vi "Main.vi"() -> ()   [LabVIEW 2020]
uses:
  Public/Controls/CCW button.ctl
  Public/Controls/CW button.ctl
  States -- typedef.ctl
  Public/Controls/Motor info.ctl
  Public/Controls/Move motor parameters--cluster.ctl
  Public/Controls/Motor direction.ctl
  Public/Controls/Step style.ctl
  Public/Controls/Com Port Options.ctl
  Public/Controls/Motor initialization parameters--cluster.ctl
  951c27e0-d3ae-4342-ab9a-27cd7722bbe2.vi
  0e09bd5c-b6a7-474e-9505-972206d0d40d.vi
  Public/Write--init.vi
  Public/Write--move.vi
  Public/Write--home.vi
  <vilib>/regexp/Match Regular Expression.xnode
  Control de MaP.lvlib
panel:
  out "Comando(string) 2":string
  in  "stop":bool
  in  "Go to zero":bool
  in  "Set zero":bool
  out "Angulo inicial":dbl caption="Ángulo \nActual M1"
  in  "Velocidad del motor\n(0-255)":u16=100
  out "Ready":bool caption="Arduino ready"
  out "Save":bool caption="Guardando datos"
  in  "Ángulo final":dbl=90.0
  out "Angulo M2":dbl caption="Ángulo \nActual M2" format="%#_3g°"
  out "Angulo M1":dbl caption="Ángulo \nActual M1" format="%#_3g°"
  out "0° M2":bool
  out "0° M1":bool
  in  "RESOLUCIÓN":dbl=1.0 caption="Avance" format="%#_g°"
  in  "CW Button M1":T1
  in  "CCW Button M1":T2
  in  "CCW Button M2":T1
  in  "CW Button M2":T2
  in  "Tab Control":T3(tab)
  out "Valor de Sensor":dbl(slide) scale=0.0..1.0
  in  "Intensidad del Láser":u8(slide) step=1 scale=0.0..255.0
  in  "Read sensor":bool
  out "Real Time Measurement":cluster{"X":dbl, "Y":dbl}[](graph)
  in  "Realizar Análisis":bool
  in  "Abrir Archivo":path
  in  "q Final":dbl=80.0
  in  "q Inicial":dbl=40.0
  out "No. de Muestras":i32
  out "Ancho de Curva":dbl format="%#.3g"
  out "Intensidad \nMáxima":dbl
  out "qR":dbl
  out "Intensidad \nMínima":dbl
  out "q Medio":dbl
  out "Brewster Angle Analysis":cluster{"EJE X":dbl[], dbl[]}(graph)
  out "Índice":dbl
  in  "Abeles Brewster":bool
  in  "Abrir Archivo de Sustrato":path
  in  "Abrir Archivo de Película":path
  in  "calcular error":bool
  out "Abeles Brewster Analysis":cluster{dbl[], dbl[]}[](graph)
  in  "q Inicial 2":dbl=40.0
  in  "q Final  2":dbl=80.0
  out "Película qB":dbl
  out "Película qB +error":dbl
  in  "Error (Grados)":dbl
  out "Sustrato qB":dbl
  out "Sustrato IR":dbl format="%#.4g"
  out "Película IR":dbl format="%#.4g"
  out "ángulo B medio":dbl
  out "Película IR +error":dbl format="%#.4g"
  in  "Home":bool
  out "Recibo de Datos":string
  in  "Get all info":bool
  in  "Read End-stops":bool
  in  "Get position":bool
  out "Idle":bool
  in  "Stop motors":bool
  in  "Move motors":bool
  # "Programa: Control de motores a pasos \npara medición de ángulo de Brewster y \ntécnica de Abelès-Brewster"
  # "Desarrollado por: Oscar Javier Silva Hernández &\nDiego Torres Armenta"
  # "Controles Manuales y Automáticos"
  # "MOTOR 1"
  # "MOTOR 2"
  # "Información del sistema"
  # "¡ATENCIÓN! Lea estas instrucciones y recomendaciones antes de operar el programa.\nEste programa ejecuta el control manual y automático del sistema en general.\nUna vez que se haya elegido el puerto COM donde tenemos ubicada nuestra tarjeta de adquisición de datos, el programa inicializará con un protocolo de calibración de motores. NO PRESIONE NINGÚN BOTÓN.\nDe manera automática el programa moverá las platinas rotatorias al ángulo 0°. Una vez que los indicadores 0° M1 y 0° M2 estén encendidos, el indicador del Ángulo Actual M1 se habilitará y el podremos iniciar a operar el programa."
  # "Controles Manuales y Automáticos (Controladores e Indicadores)\n\n-MOTOR 1 & 2: Para ambos motores se tiene un botón de movimiento hacia adelante y otro botón de movimiento hacia atrás indicado con flechas. Durante el reinicio de posición 0°, el botón hacia atrás se deshabilita para evitar conflictos mecánicos.\n-0° M1 & 0° M2: Indicadores de posición 0° para ambos motores.\n-FIN: Indica si se está terminó de realizar un movimiento.\n-Ángulo Actual M1 & M2: Muestra la posición actual para cada motor.\n-RESOLUCIÓN: Valor de grados definido por el usuario para realizar movimientos manuales de manera independiente para cada motor. Es utilizado para alinear el sistema con respecto al láser antes y después de realizar mediciones.\n-Reiniciar Posición: Inicia el protocolo de reinicio de posición para regresar los motores a 0°.\n-Mover y Guardar: Se inicia el barrido ángular desde la posición actual de los motores hasta la posición indicada en el controlador Barrido Angular.\n-Cancelar: Cancela cualquier movimiento o instrucción que se esté ejecutando. My útil para detener instrucciones y cerrar el programa sin tener conflictos."
  # "Parámetros iniciales & Información (Controladores e Indicadores)\n\n-SALIR: Cerramos el programa una vez que hayamos terminado de utilizarlo. Es importante no presionar este botón en medio de un movimiento de motor o alguna otra instrucción.\n-Pantalla: Toda la información generada por los eventos de usuario es mostrada en esta pantalla.\n-Programa habilitado: Se enciende cuando el proceso de inicialización se realiza exitosamente y el programa queda listo para operar.\n-Guardar Datos: Indica si los datos están siendo capturados durante el barrido angular."
  # "Gráfica, Ángulo de Brewster & Abelès-Brewster Analysis\n\n-Gráfica: Esta sección es utilizada para llevar a cabo las mediciones. Dentro podemos encontrar un indicador del valor de la intensidad de la luz capturada por el sensor, un controlador para la intensidad de la luz de salida del láser semiconductor.\n-Ángulo de Brewster: En esta sección podemos realizar el análisis de ángulo de Brewster de mediciones realizadas por el sistema para encontrar los parámetros característicos de la curva. Seleccionamos el archivo deseado, definimos el ángulo inicial y final y presionamos el botón ANALISIS.\n-Abelès-Brewster: Muy similar a la sección anterior, podemos realizar el ánalisis de Abelès-Brewster de mediciones realizadas para sustratos con y sin película delgada. También podemos calcular el error del resultado."
  # "Montura de\nSustratos"
  # "Ensamble \nde Motores"
  # "Montura \nde Prismas"
  # "Sistema Completo con Montura de Sustratos"
  # "Ensamble de Láser con Polarizador"
  # "Sistema Completo con Montura de Prismas"
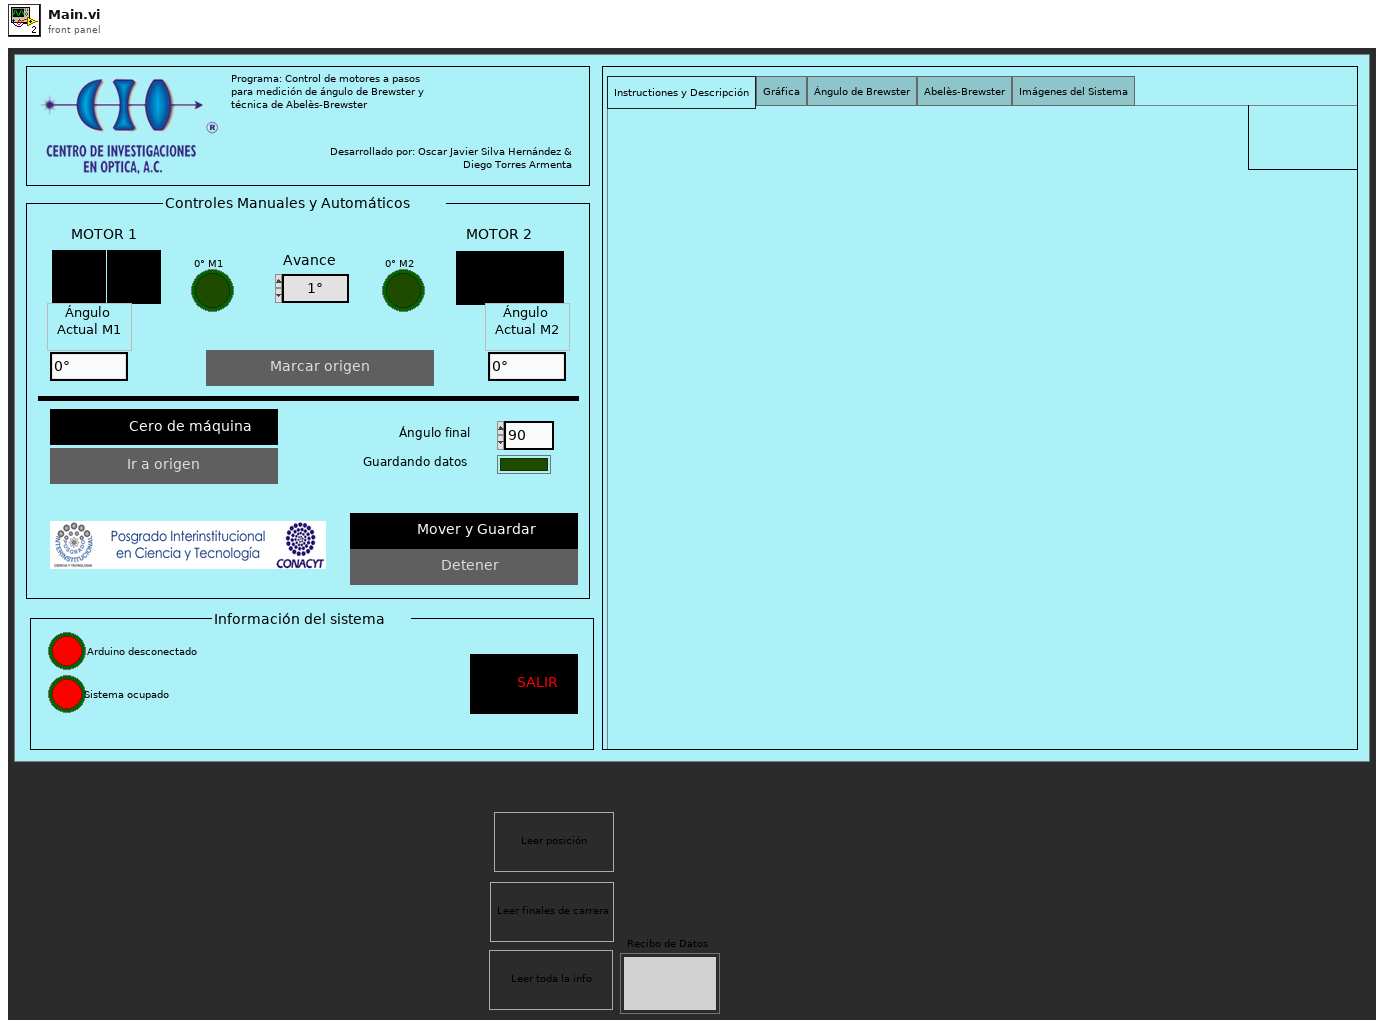
[diagram p1: front panel]
types:
  T1 = typedef "CW button.ctl" = bool
  T2 = typedef "CCW button.ctl" = bool
  T3 = enum32{"Instructiones y Descripción", "Gráfica", "Ángulo de Brewster", "Abelès-Brewster", "Imágenes del Sistema"}
  T4 = cluster{"refnum out":refnum<file>, "path":path, "path string":string}
  T5 = typedef "Control de MaP.lvlib/Motor info.ctl" = cluster{"Motor positions":dbl[], "Sensor value":dbl, "End-stop state":bool[], "°/step":dbl[], "Motor params":T6, "Moving?":bool, "Home?":bool, "Connected?":bool, "Manual zero?":bool}
  T6 = typedef "Control de MaP.lvlib/Move motor parameters--cluster.ctl" = cluster{"Action":u8, "Direction motor 1":T7, "Direction motor 2":T7, "Steps motor 1":u16, "Steps motor 2":u16, "Step style motor 1":T8, "Step style motor 2":T8}
  T7 = typedef "Control de MaP.lvlib/Motor direction.ctl" = u8
  T8 = typedef "Control de MaP.lvlib/Step style.ctl" = u8
  T9 = typedef "States -- typedef.ctl" = enum16{"Initilaize", "Update FP", "Enable/disable controls", "Wait", "Update config", "Configuration dialog", "Exit", "Init motor"}
  T10 = typedef "Config -- cluster.ctl" = cluster{"Arduino port":refnum<visa-resource-name>, "Starting angle M1":dbl, "Starting angle M2":dbl}
  T11 = enum8{"Enabled", "Disabled", "Disabled and Grayed Out"}
  T12 = typedef "Control de MaP.lvlib/Motor initialization parameters--cluster.ctl" = cluster{"Action":u8, "Steps per rev motor 1":u8, "Steps per rev motor 2":u8, "RPM motor 1":u16, "RPM motor 2":u16}
  T13 = typedef "Control de MaP.lvlib/Com Port Options.ctl" = cluster{"baud rate (9600)":u32, "data bits (8)":u16, "parity (0:none)":enum16{"None", "Odd", "Even", "Mark", "Space"}}
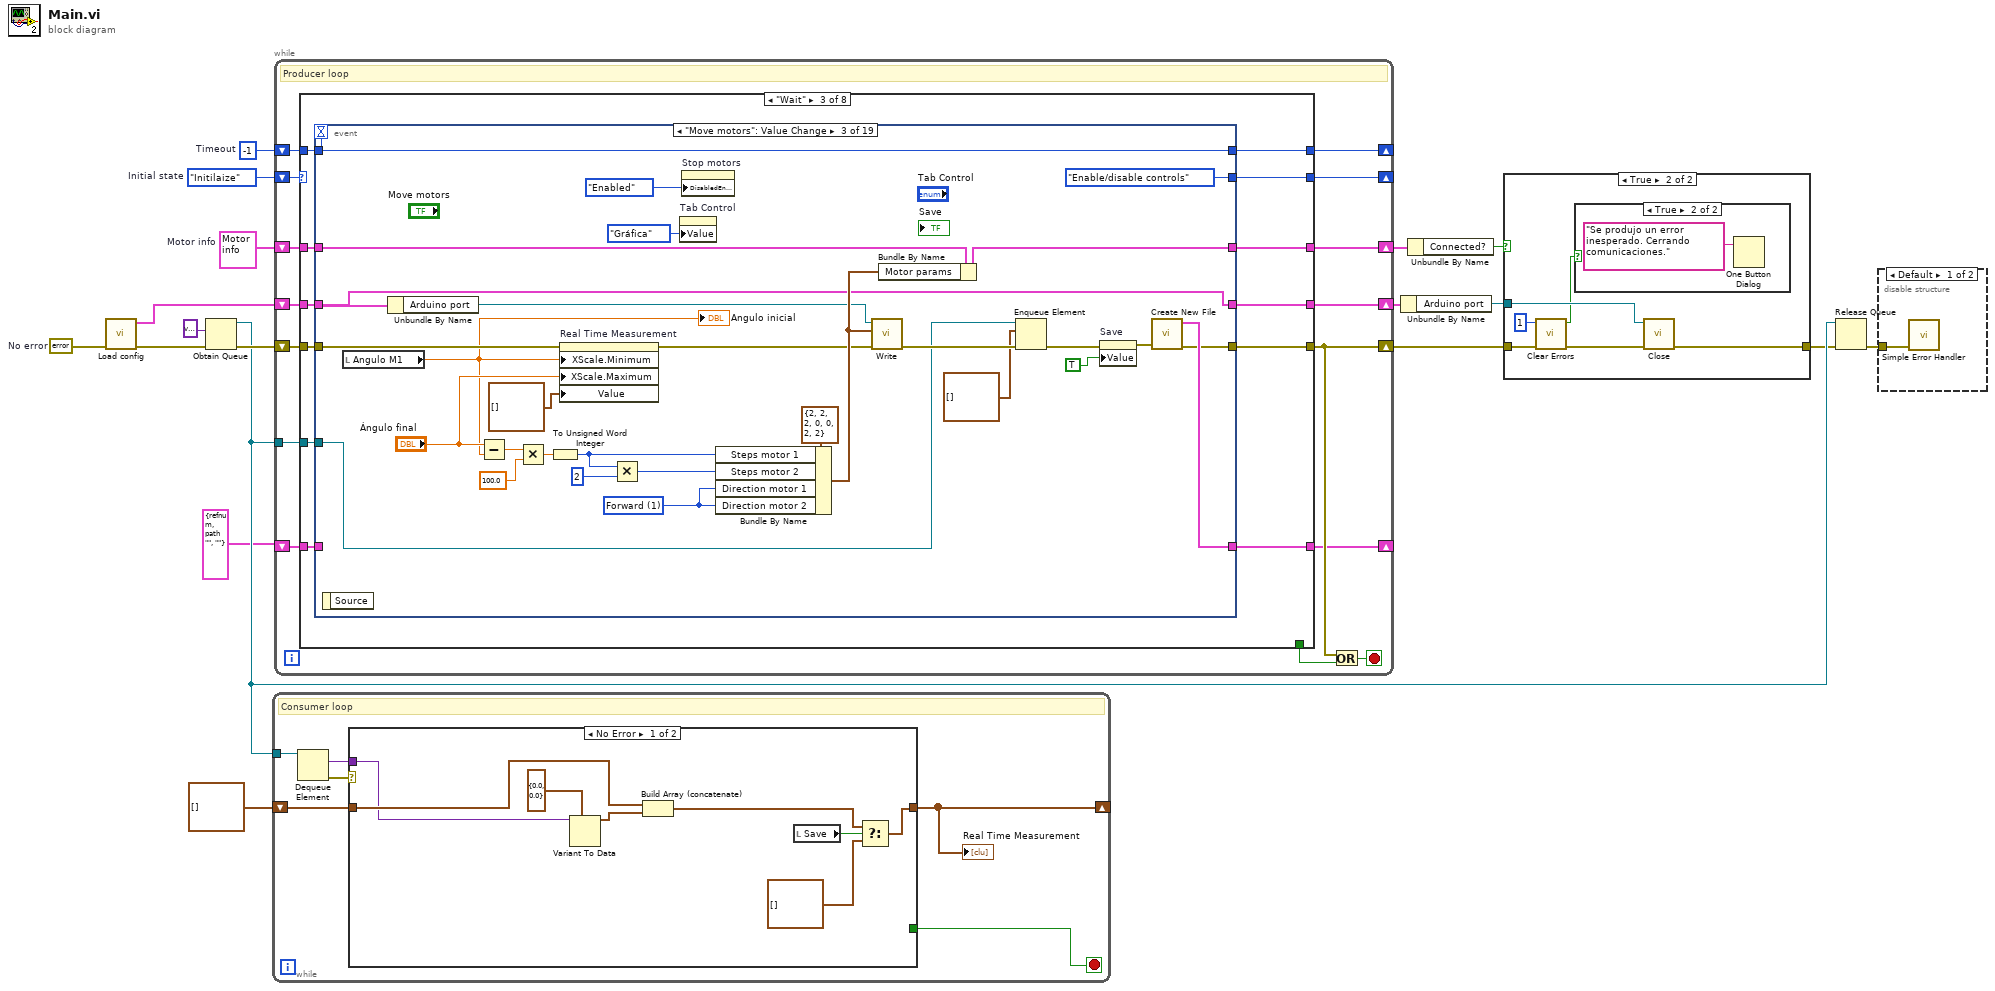
[diagram p0: block diagram]
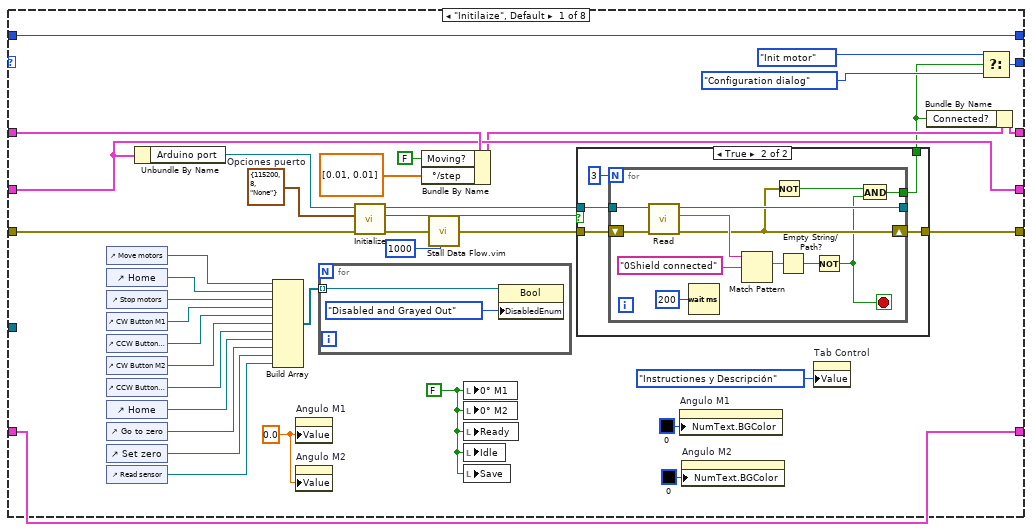
[diagram p2: hidden frame]
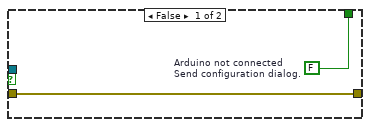
[diagram p3: hidden frame]
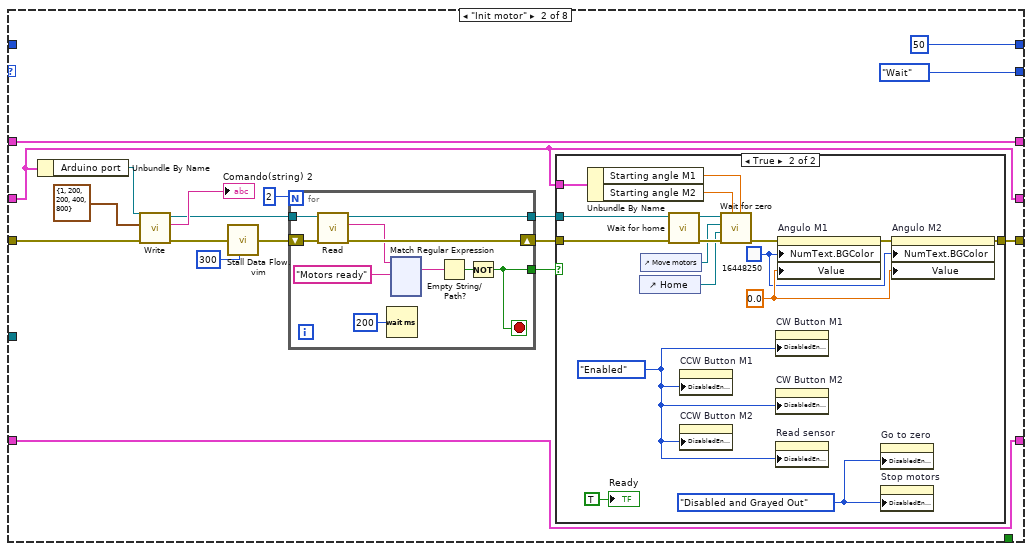
[diagram p4: hidden frame]
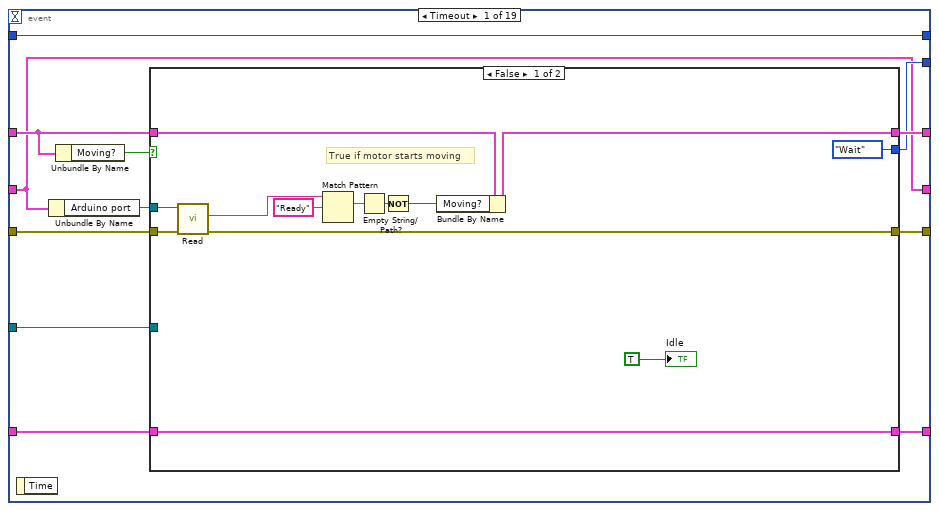
[diagram p6: hidden frame]
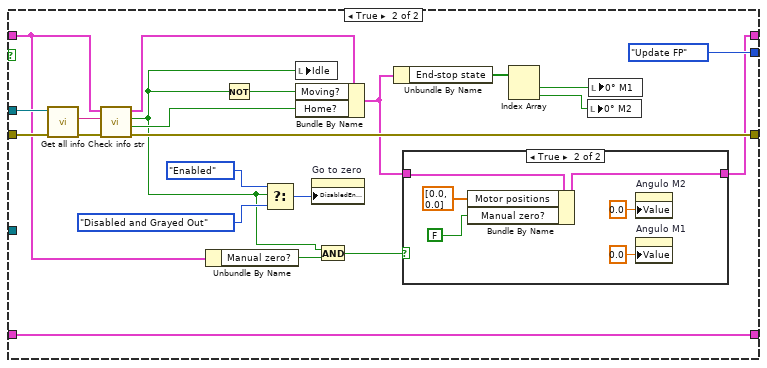
[diagram p7: hidden frame]
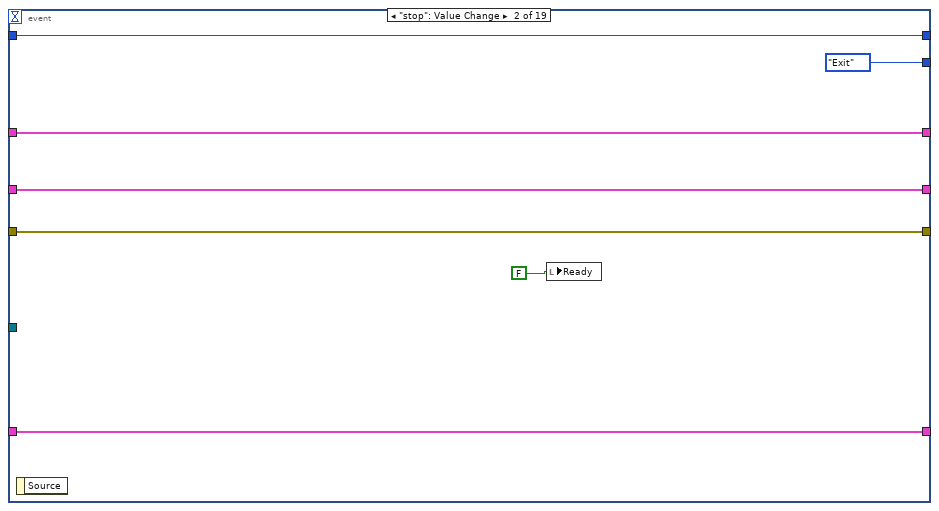
[diagram p9: hidden frame]
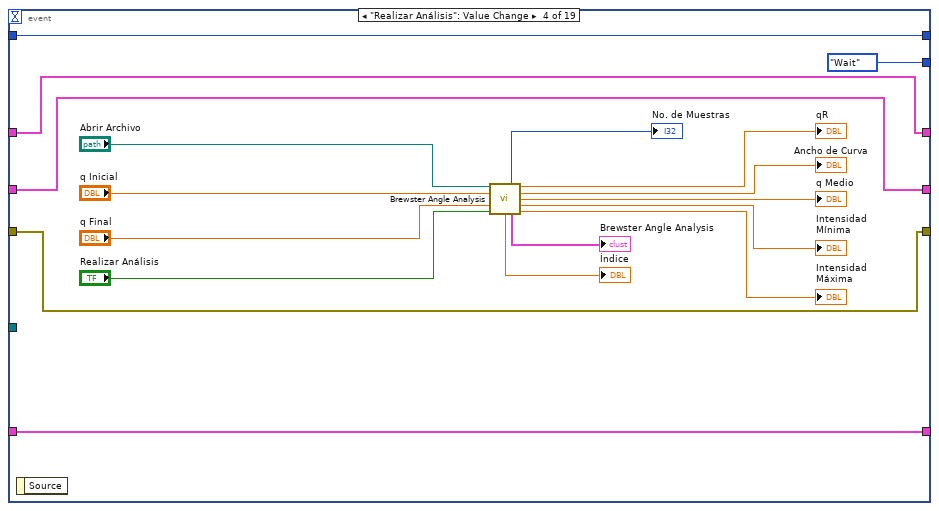
[diagram p10: hidden frame]
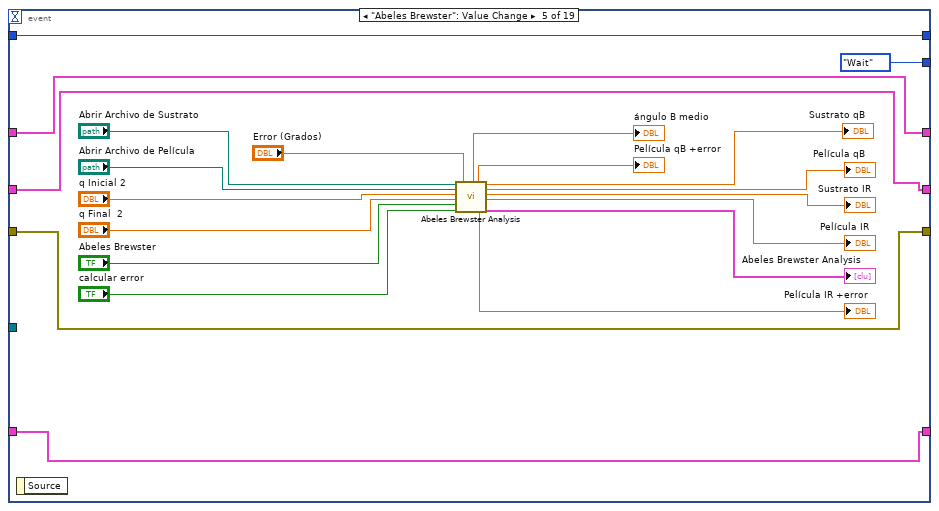
[diagram p11: hidden frame]
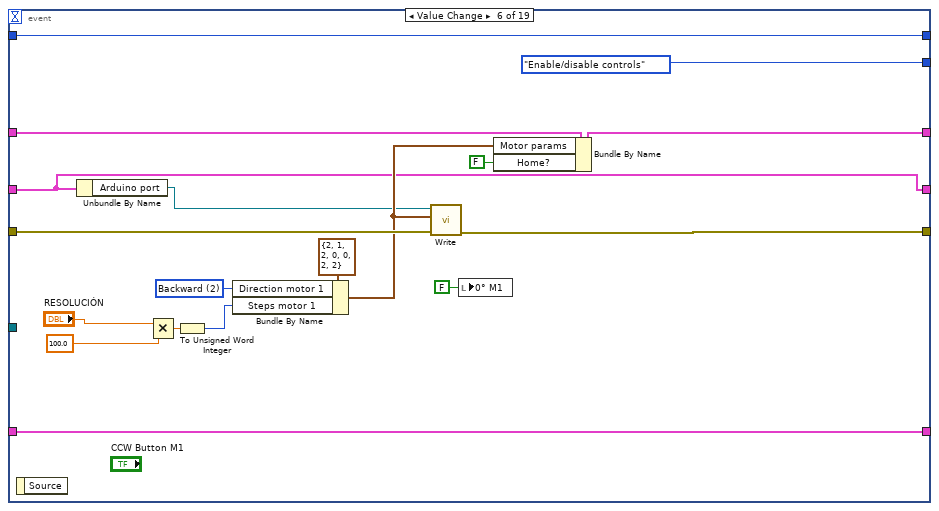
[diagram p12: hidden frame]
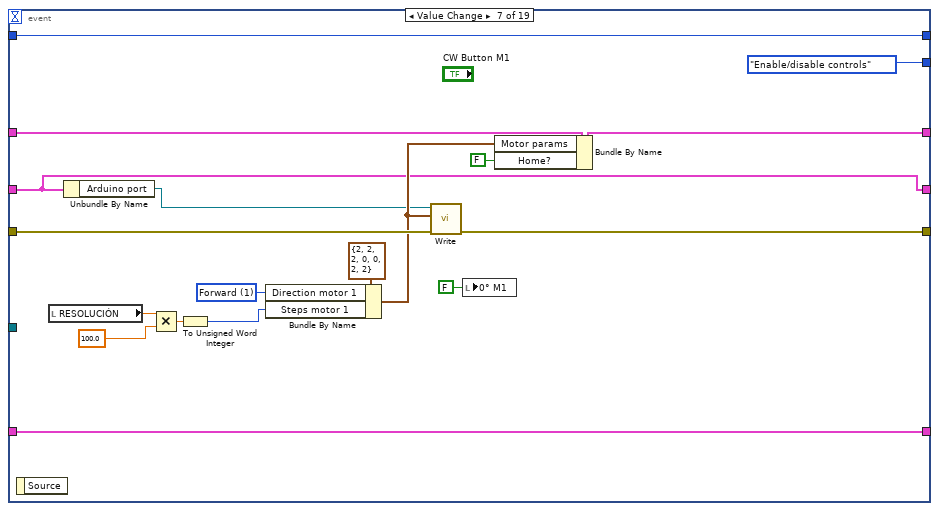
[diagram p13: hidden frame]
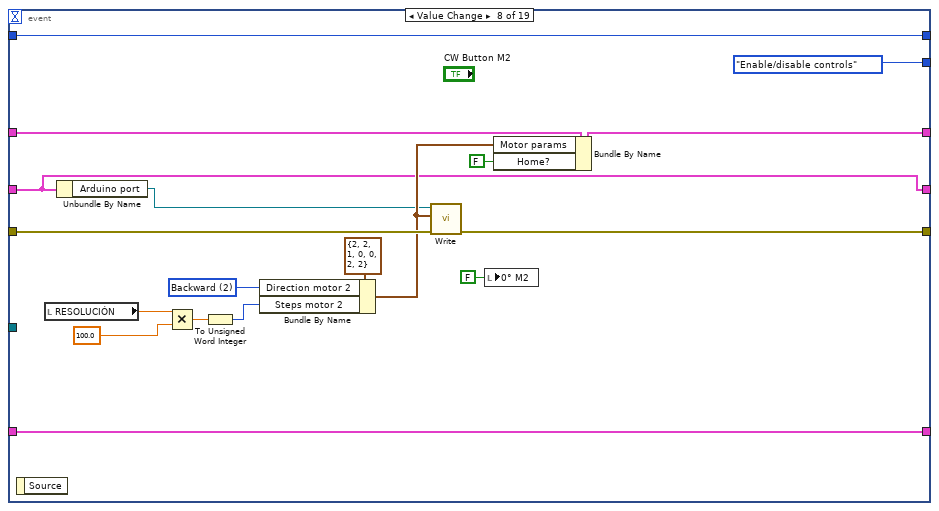
[diagram p14: hidden frame]
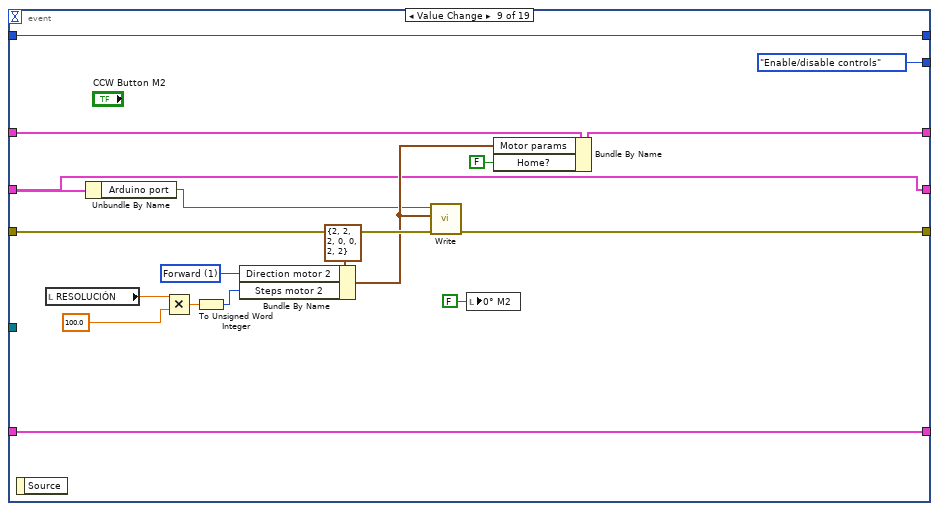
[diagram p15: hidden frame]
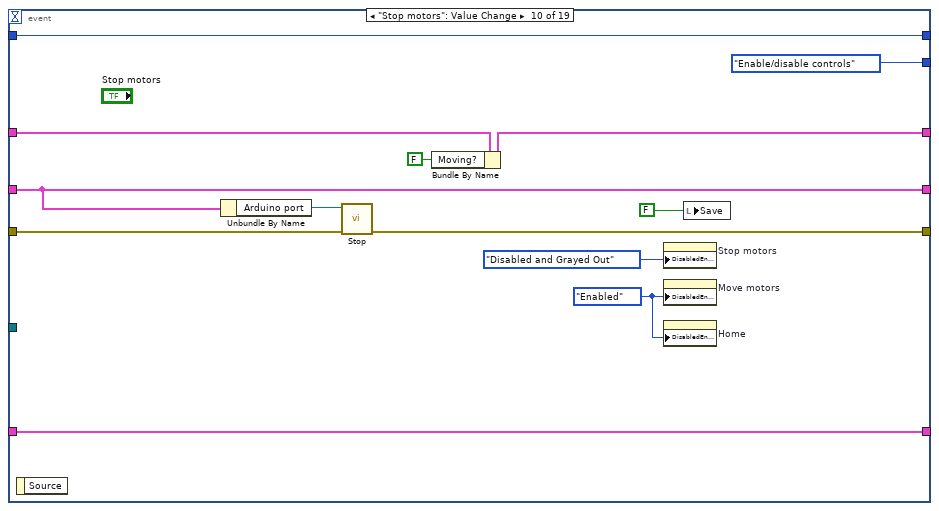
[diagram p16: hidden frame]
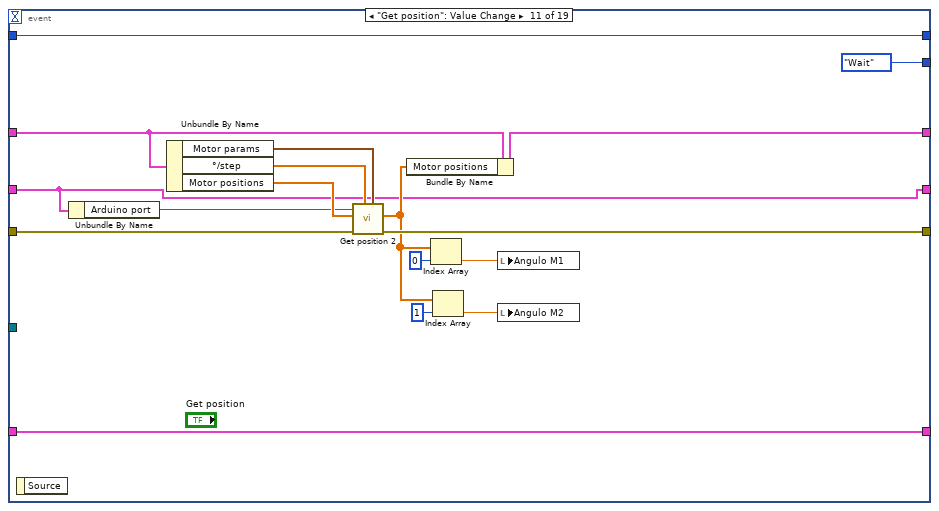
[diagram p17: hidden frame]
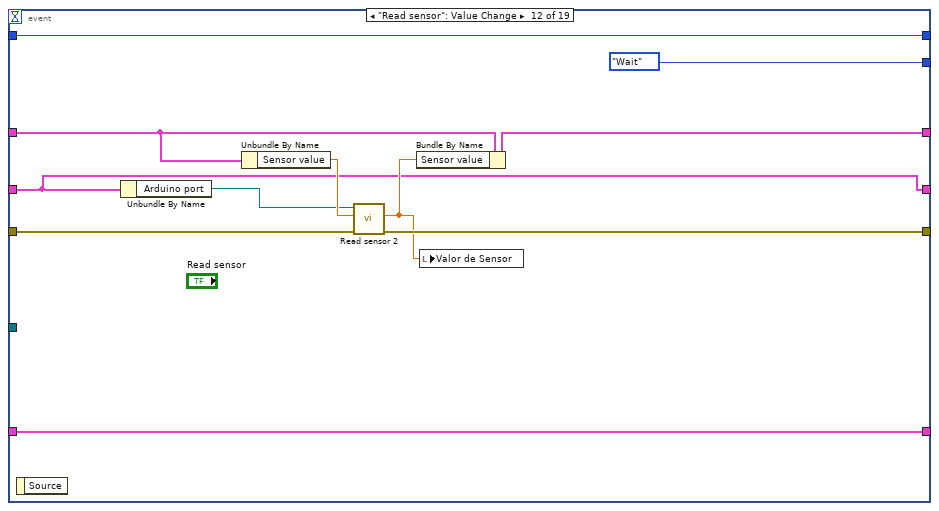
[diagram p18: hidden frame]
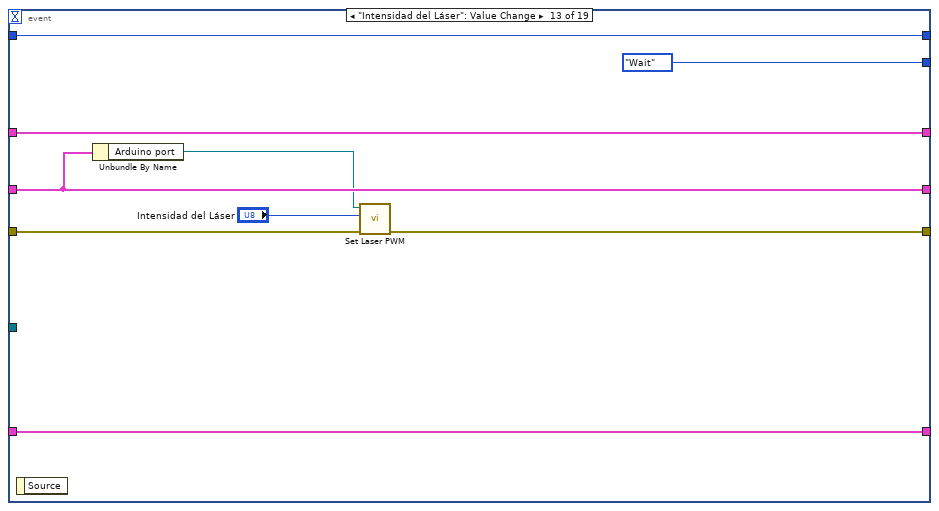
[diagram p19: hidden frame]
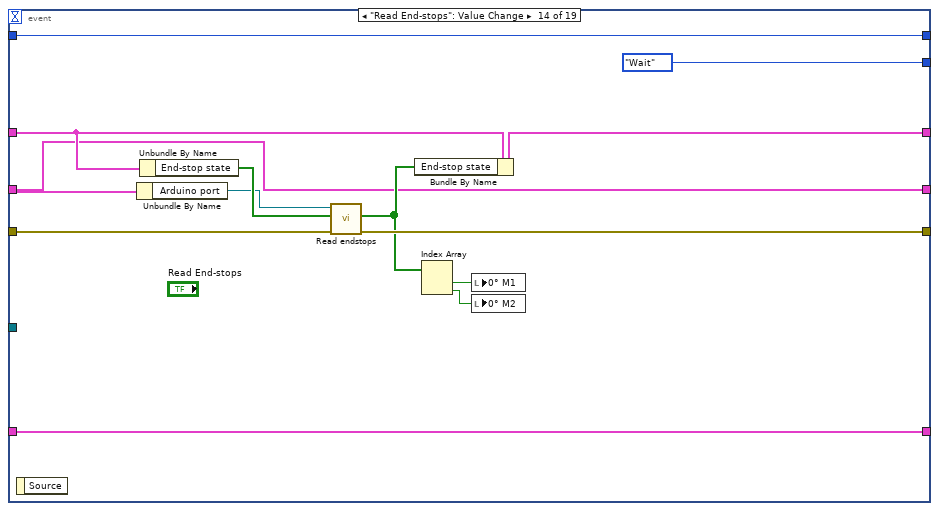
[diagram p20: hidden frame]
diagram:
  w15 = T5 {"Motor positions"=[0.0, 0.0], "Sensor value"=0.0, "End-stop state"=[FALSE, FALSE], "°/step"=[], "Motor params"={"Action"=2, "Direction motor 1"=1, "Direction motor 2"=1, "Steps motor 1"=100, "Steps motor 2"=100, "Step style motor 1"=1, "Step style motor 2"=1}, "Moving?"=FALSE, "Home?"=FALSE, "Connected?"=FALSE, "Manual zero?"=FALSE}  # Motor info
  w16 = -1  # Timeout
  w4 = errorcluster {"status"=FALSE, "code"=0, "source"=""}  # No error
  w18 = States_--_typedef."Initilaize"  # Initial state
  n1 = call "Load config.vi"("error in (no error)"=w4) -> ("error out"=w3:errorcluster, "Config"=w5:T10)  [unwired: 9 in]
  n2 = Obtain Queue(element data type=variant, error in (no error)=w3) -> (queue out=w11:refnum<queue>, error out=w13:errorcluster)  [unwired: 3 in, 1 out]
  n3 = while {
    tunnel: w11 -> [w24]
    shift-right: [w19] -> _
    shift-left: cluster{"Ángulo M1":dbl, "Voltage":dbl}[] [] ("cluster") -> [w23]
    stop <- w20 stop-if-true
    # "Consumer loop"
    n4 = Dequeue Element(queue=w24) -> (element=w22:variant, error out=w21:errorcluster)  [unwired: 2 in, 2 out]
    n5 = case shown="No Error" w21 {
      tunnel: w23 -> [w32 _]
      tunnel: w22 -> [w31 _]
      tunnel: [w26 cluster{"Ángulo M1":dbl, "Voltage":dbl}[] [] ("cluster")] -> w19
      tunnel: [_ TRUE] -> w20
      frame No Error {
        n6 = Variant To Data(type=cluster{"Ángulo M1":dbl, "Voltage":dbl} {"Ángulo M1"=0.0, "Voltage"=0.0} ("cluster"), Variant=w31) -> (data=w29:cluster{"Ángulo M1":dbl, "Voltage":dbl})  [unwired: 1 in, 1 out]
        n7 = Build Array (concatenate)(w32, w29) -> (w28:cluster{"Ángulo M1":dbl, "Voltage":dbl}[])
        n8 = local read "Save"() -> (w25:bool)
        n9 = Select(t=w28, s=w25, f=cluster{"Ángulo M1":dbl, "Voltage":dbl}[] [] ("cluster")) -> (s? t:f=w26:cluster{"Ángulo M1":dbl, "Voltage":dbl}[])
      }
      frame Error {
      }
    }
    "Real Time Measurement" <- w19
  }
  n10 = while {
    shift-right: [w48] -> _
    shift-left: w18 -> [w49]
    shift-right: [w45] -> w17
    shift-left: w13 -> [w47]
    shift-right: [w43] -> _
    shift-left: w16 -> [w44]
    shift-right: [w41] -> w2
    shift-left: w15 -> [w42]
    tunnel: w11 -> [w40]
    shift-right: [w38] -> _
    shift-left: T4 {"refnum out"=refnum, "path"=path "", "path string"=""} ("File Directory") -> [w37]
    shift-right: [w36] -> w7
    shift-left: w5 -> [w35]
    stop <- w39 stop-if-true
    # "Producer loop"
    n11 = case shown="\"Wait\"" w49 {
      tunnel: [_ _ _ _ _ _ _ "stop"] -> w46
      tunnel: [w72 States_--_typedef."Wait" ("Unused") w280 w645 States_--_typedef."Wait" ("Unused") States_--_typedef."Enable/disable controls" ("Unused") States_--_typedef."Wait" ("Unused") w735] -> w48
      tunnel: [w74 w112 w279 w650 w672 w692 w719 w732] -> w45
      tunnel: w47 -> [w87 w125 w278 w651 w673 w690 w719 w733]
      tunnel: w44 -> [w85 _ w276 w654 w674 w698 w718 w734]
      tunnel: [w85 50 ("Timeout") w277 w654 w674 w698 w718 w734] -> w43
      tunnel: w42 -> [w84 w110 w275 w653 w666 w697 w715 w729]
      tunnel: [w55 w110 w274 w653 w665 w697 w715 w729] -> w41
      tunnel: w40 -> [_ _ w273 _ _ w675 _ _]
      tunnel: [w78 w126 w272 w652 w670 w693 w717 w731] -> w38
      tunnel: w37 -> [w78 w126 w271 w652 w670 w693 w717 w731]
      tunnel: [w70 w109 w269 w648 w671 w689 w712 w730] -> w36
      tunnel: w35 -> [w70 w109 w270 w647 w671 w689 w712 w730]
      frame "Initilaize", Default {
        w52 = 0.0 ("Angulo M1")
        w65 = FALSE ("0° M1")
        w86 = T13 {"baud rate (9600)"=115200, "data bits (8)"=8, "parity (0:none)"=enum."None"}  # Opciones puerto
        n12 = control-ref of="Move motors"() -> (w81:refnum<vi>)
        n13 = control-ref of="Home"() -> (w80:refnum<vi>)
        n14 = control-ref of="Stop motors"() -> (w79:refnum<vi>)
        n15 = control-ref of="CW Button M1"() -> (w64:refnum<vi>)
        n16 = control-ref of="CCW Button M1"() -> (w63:refnum<vi>)
        n17 = control-ref of="CW Button M2"() -> (w62:refnum<vi>)
        n18 = control-ref of="CCW Button M2"() -> (w61:refnum<vi>)
        n19 = control-ref of="Home"() -> (w60:refnum<vi>)
        n20 = control-ref of="Go to zero"() -> (w59:refnum<vi>)
        n21 = control-ref of="Set zero"() -> (w58:refnum<vi>)
        n22 = control-ref of="Read sensor"() -> (w53:refnum<vi>)
        n23 = Unbundle By Name(w70) -> ("Arduino port"=w69:refnum<visa-resource-name>)
        n24 = Build Array(w81, w80, w79, w64, w63, w62, w61, w60, w59, w58, w53) -> (w82:refnum<vi>[])
        n25 = property on="Angulo M1" class="DigNum (strict)"("Value"=w52) -> ()  [unwired: 2 in, 2 out]
        n26 = property on="Angulo M2" class="DigNum (strict)"("Value"=w52) -> ()  [unwired: 2 in, 2 out]
        n27 = for {
          tunnel: w82 -> [w107] mode=indexing
          n28 = property class="Bool"(reference=w107, "DisabledEnum"=T11."Disabled and Grayed Out" ("Disabled")) -> ()  [unwired: 1 in, 2 out]
        }
        n29 = call "Initialize.vi"("error in (no error)"=w87, "Opciones puerto"=w86, "Puerto Serial"=w69) -> ("error out"=w76:errorcluster, "Connected?"=w57:bool, "VISA resource name out"=w75:refnum<visa-resource-name>)  [unwired: 6 in]
        n30 = Bundle By Name(cluster=w84, "Moving?"=FALSE, "°/step"=dbl[] [0.01, 0.01]) -> (w56:T5)
        n31 = call "Stall Data Flow.vim"("value in"=w76, "milliseconds to wait"=u32 1000) -> ("value out"=w67:errorcluster)  [unwired: 1 out]
        n32 = local write "0° M1"(w65) -> ()
        n33 = local write "0° M2"(w65) -> ()
        n34 = local write "Ready"(w65) -> ()
        n35 = local write "Idle"(w65) -> ()
        n36 = local write "Save"(w65) -> ()
        n37 = case shown="True" w57 {
          tunnel: w75 -> [_ w94]
          tunnel: [w89 w93] -> w74
          tunnel: [w88 w92] -> w54
          tunnel: w67 -> [w89 w90]
          frame False {
            w88 = FALSE  # Arduino not connected Send configuration dialog.
          }
          frame True {
            n38 = for {
              N: 3 -> [_]
              shift-right: [w99] -> w93
              shift-left: w90 -> [w106]
              tunnel: [w96] -> w92
              tunnel: w94 -> [w105]
              tunnel: [w104] -> _
              stop <- w95 stop-if-true
              n39 = call "Read.vi"("error in (no error)"=w106, "VISA resource name"=w105) -> ("error out"=w99:errorcluster, "Recibo de Datos"=w101:string, "VISA resource name out"=w104:refnum<visa-resource-name>)  [unwired: 6 in, 1 out]
              n40 = Wait (ms)(milliseconds to wait=u32 200) -> ()  [unwired: 1 out]
              n41 = Match Pattern(string=w101, regular expression="0Shield connected") -> (match substring=w103:string)  [unwired: 1 in, 3 out]
              n42 = Not(x=w99) -> (.not. x?=w97:bool)
              n43 = Empty String/Path?(string/path=w103) -> (empty?=w98:bool)
              n44 = Not(x=w98) -> (.not. x?=w95:bool)
              n45 = And(x=w97, y=w95) -> (x .and. y?=w96:bool)
            }
          }
        }
        n46 = property on="Angulo M1" class="DigNum (strict)"("NumText.BGColor"=u32 0 ("Caption.Colors:BG Color")) -> ()  [unwired: 2 in, 2 out]
        n47 = property on="Angulo M2" class="DigNum (strict)"("NumText.BGColor"=u32 0 ("Caption.Colors:BG Color")) -> ()  [unwired: 2 in, 2 out]
        n48 = property on="Tab Control" class="TabCtl (strict)"("Value"=T3."Instructiones y Descripción" ("Tab Control")) -> ()  [unwired: 2 in, 2 out]
        n49 = Bundle By Name(cluster=w56, "Connected?"=w54) -> (w55:T5)
        n50 = Select(t=States_--_typedef."Init motor" ("Unused"), s=w54, f=States_--_typedef."Configuration dialog") -> (s? t:f=w72:T9)
      }
      frame "Init motor" {
        n51 = Unbundle By Name(w109) -> ("Arduino port"=w124:refnum<visa-resource-name>)
        n52 = call-poly "Write.vi"("error in (no error)"=w125, "Comando"=T12 {"Action"=1, "Steps per rev motor 1"=200, "Steps per rev motor 2"=200, "RPM motor 1"=400, "RPM motor 2"=800}, "VISA resource name"=w124) -> ("error out"=w120:errorcluster, "Comando(string)"=→"Comando(string) 2":string, "VISA resource name out"=w119:refnum<visa-resource-name>)  [unwired: 6 in]
        n53 = call "Stall Data Flow.vim"("value in"=w120, "milliseconds to wait"=u32 300) -> ("value out"=w118:errorcluster)  [unwired: 1 out]
        n54 = for {
          N: 2 -> [_]
          tunnel: w119 -> [w153]
          shift-right: [w152] -> w113
          shift-left: w118 -> [w149]
          tunnel: [w146] -> w114
          tunnel: [w145] -> w111
          stop <- w146 stop-if-true
          n55 = call "Read.vi"("error in (no error)"=w149, "VISA resource name"=w153) -> ("error out"=w152:errorcluster, "Recibo de Datos"=w151:string, "VISA resource name out"=w145:refnum<visa-resource-name>)  [unwired: 6 in, 1 out]
          n56 = Wait (ms)(milliseconds to wait=u32 200) -> ()  [unwired: 1 out]
          n57 = xnode "Match Regular Expression"("input string"=w151, "regular expression"="Motors ready") -> ("whole match"=w150:string)  [unwired: 4 in, 4 out]
          n58 = Empty String/Path?(string/path=w150) -> (empty?=w148:bool)
          n59 = Not(x=w148) -> (.not. x?=w146:bool)
        }
        n60 = case shown="True" w114 {
          tunnel: w113 -> [w127 w144]
          tunnel: [w127 w130] -> w112
          tunnel: w111 -> [_ w143]
          tunnel: w109 -> [_ w140]
          frame False {
          }
          frame True {
            w128 = u32 16448250 ("Caption.Colors:BG Color")
            w129 = 0.0 ("Angulo M1")
            w137 = T11."Enabled" ("Disabled")
            w136 = T11."Disabled and Grayed Out" ("Disabled")
            n61 = Unbundle By Name(w140) -> ("Starting angle M1"=w138:dbl, "Starting angle M2"=w139:dbl)
            n62 = control-ref of="Home"() -> (w134:refnum<vi>)
            n63 = control-ref of="Move motors"() -> (w135:refnum<vi>)
            n64 = call "Wait for home.vi"("error in (no error)"=w144, "VISA Refnum in"=w143) -> ("error out"=w142:errorcluster, "VISA resource name out"=w141:refnum<visa-resource-name>)  [unwired: 8 in]
            n65 = property on="CCW Button M1" class="Bool"("DisabledEnum"=w137) -> ()  [unwired: 2 in, 2 out]
            n66 = property on="CCW Button M2" class="Bool"("DisabledEnum"=w137) -> ()  [unwired: 2 in, 2 out]
            n67 = call "Wait for zero.vi"("Starting angle M1"=w138, "Starting angle M2"=w139, "error in (no error)"=w142, "Home ctrl ref"=w134, "Move motor ctrl ref"=w135, "VISA resource name"=w141) -> ("error out"=w132:errorcluster)  [unwired: 5 in]
            n68 = property on="CW Button M1" class="Bool"("DisabledEnum"=w137) -> ()  [unwired: 2 in, 2 out]
            n69 = property on="CW Button M2" class="Bool"("DisabledEnum"=w137) -> ()  [unwired: 2 in, 2 out]
            n70 = property on="Read sensor" class="Bool"("DisabledEnum"=w137) -> ()  [unwired: 2 in, 2 out]
            n71 = property on="Angulo M1" class="DigNum (strict)"(error in=w132, "NumText.BGColor"=w128, "Value"=w129) -> (error out=w131:errorcluster)  [unwired: 1 in, 1 out]
            n72 = property on="Go to zero" class="Bool"("DisabledEnum"=w136) -> ()  [unwired: 2 in, 2 out]
            n73 = property on="Stop motors" class="Bool"("DisabledEnum"=w136) -> ()  [unwired: 2 in, 2 out]
            n74 = property on="Angulo M2" class="DigNum (strict)"(error in=w131, "NumText.BGColor"=w128, "Value"=w129) -> (error out=w130:errorcluster)  [unwired: 1 in, 1 out]
            "Ready" <- TRUE ("Ready")
          }
        }
      }
      frame "Wait" {
        n75 = event shown="[2] \"Move motors\": Value Change" {
          selector: _ -> [_ _ _ _ _ _ _ _ _ _ _ _ _ _ _ _ _ _ _]
          dyn-events: _ -> [_ _ _ _ _ _ _ _ _ _ _ _ _ _ _ _ _ _ _]
          timeout: w276 -> [_ _ _ _ _ _ _ _ _ _ _ _ _ _ _ _ _ _ _]
          tunnel: [w283 States_--_typedef."Exit" ("Unused") States_--_typedef."Enable/disable controls" ("Unused") States_--_typedef."Wait" ("Unused") States_--_typedef."Wait" ("Unused") States_--_typedef."Enable/disable controls" ("Unused") States_--_typedef."Enable/disable controls" ("Unused") States_--_typedef."Enable/disable controls" ("Unused") States_--_typedef."Enable/disable controls" ("Unused") States_--_typedef."Enable/disable controls" ("Unused") States_--_typedef."Wait" ("Unused") States_--_typedef."Wait" ("Unused") States_--_typedef."Wait" ("Unused") States_--_typedef."Wait" ("Unused") States_--_typedef."Wait" ("Unused") States_--_typedef."Wait" ("Unused") States_--_typedef."Wait" ("Unused") States_--_typedef."Update config" ("Unused") States_--_typedef."Enable/disable controls" ("Unused")] -> w280
          tunnel: [w291 w340 w358 w389 w410 w428 w446 w464 w482 w495 w509 w520 w530 w544 w553 w563 w577 w593 w623] -> w279
          tunnel: w278 -> [w292 w340 w357 w389 w410 w426 w444 w462 w480 w494 w512 w523 w531 w543 w555 w560 w578 w593 w599]
          tunnel: [w287 w339 w368 w388 w409 w423 w441 w459 w477 w487 w511 w522 w532 w545 w556 w569 w583 w596 w634] -> w277
          tunnel: w276 -> [w287 w339 w368 w388 w409 w423 w441 w459 w477 w487 w511 w522 w532 w545 w556 w569 w583 w596 w634]
          tunnel: w275 -> [w289 w338 w370 w387 w408 w425 w443 w461 w479 w492 w507 w518 w529 w541 w551 w562 w582 w591 w603]
          tunnel: [w290 w338 w369 w387 w408 w424 w442 w460 w478 w491 w506 w517 w529 w540 w550 w565 w582 w591 w602] -> w274
          tunnel: w273 -> [w286 _ w343 _ _ _ _ _ _ _ _ _ _ _ _ _ _ _ _]
          tunnel: [w284 w336 w359 w373 w391 w416 w434 w452 w470 w485 w499 w515 w526 w536 w548 w568 w581 w595 w633] -> w272
          tunnel: w271 -> [w285 w336 _ w373 w391 w416 w434 w452 w470 w485 w499 w515 w526 w536 w548 w568 w581 w595 w633]
          tunnel: w270 -> [w282 w335 w354 w372 w390 w414 w432 w450 w468 w484 w497 w514 w525 w534 w547 w564 w575 w590 w632]
          tunnel: [w282 w335 w354 w372 w390 w414 w432 w450 w468 w484 w497 w514 w525 w534 w547 w564 w575 w592 w632] -> w269
          event Timeout {
            n76 = event-data() -> ()  [unwired: 1 in, 1 out]
            n77 = Unbundle By Name(w282) -> ("Arduino port"=w281:refnum<visa-resource-name>)
            n78 = Unbundle By Name(w289) -> ("Moving?"=w288:bool)
            n79 = case shown="False" w288 {
              tunnel: w292 -> [w305 w327]
              tunnel: [w297 w323] -> w291
              tunnel: w281 -> [w304 w326]
              tunnel: w289 -> [w302 w309]
              tunnel: [w301 w310] -> w290
              tunnel: w286 -> [_ _]
              tunnel: w285 -> [w298 w320]
              tunnel: [w298 w320] -> w284
              tunnel: [States_--_typedef."Wait" ("Unused") States_--_typedef."Update FP" ("Unused")] -> w283
              frame False {
                # "True if motor starts moving"
                n80 = call "Read.vi"("error in (no error)"=w305, "VISA resource name"=w304) -> ("error out"=w297:errorcluster, "Recibo de Datos"=w294:string)  [unwired: 6 in, 2 out]
                n81 = Match Pattern(string=w294, regular expression="Ready") -> (match substring=w299:string)  [unwired: 1 in, 3 out]
                n82 = Empty String/Path?(string/path=w299) -> (empty?=w300:bool)
                n83 = Not(x=w300) -> (.not. x?=w295:bool)
                n84 = Bundle By Name(cluster=w302, "Moving?"=w295) -> (w301:T5)
                "Idle" <- TRUE ("READY")
              }
              frame True {
                n85 = call "Get all info.vi"("error in (no error)"=w327, "VISA Refnum in"=w326) -> ("error out"=w325:errorcluster, "Recibo de Datos"=w316:string)  [unwired: 7 in, 1 out]
                n86 = call "Check info str.vi"("error in (no error)"=w325, "Data in"=w316, "Motor info"=w309) -> ("error out"=w323:errorcluster, "Home?"=w315:bool, "End?"=w306:bool, "Motor info out"=w324:T5)  [unwired: 5 in]
                n87 = Unbundle By Name(w309) -> ("Manual zero?"=w307:bool)
                n88 = Not(x=w306) -> (.not. x?=w322:bool)
                n89 = Select(t=T11."Enabled" ("Disabled"), s=w306, f=T11."Disabled and Grayed Out") -> (s? t:f=w312:T11)
                n90 = local write "Idle"(w306) -> ()
                n91 = Bundle By Name(cluster=w324, "Moving?"=w322, "Home?"=w315) -> (w311:T5)
                n92 = property on="Go to zero" class="Bool"("DisabledEnum"=w312) -> ()  [unwired: 2 in, 2 out]
                n93 = And(x=w306, y=w307) -> (x .and. y?=w308:bool)
                n94 = Unbundle By Name(w311) -> ("End-stop state"=w319:bool[])
                n95 = case shown="True" w308 {
                  tunnel: w311 -> [w328 w332]
                  tunnel: [w328 w331] -> w310
                  frame False {
                  }
                  frame True {
                    n96 = Bundle By Name(cluster=w332, "Motor positions"=dbl[] [0.0, 0.0], "Manual zero?"=FALSE) -> (w331:T5)
                    n97 = property on="Angulo M2" class="DigNum (strict)"("Value"=0.0 ("Angulo M2")) -> ()  [unwired: 2 in, 2 out]
                    n98 = property on="Angulo M1" class="DigNum (strict)"("Value"=0.0 ("Angulo M1")) -> ()  [unwired: 2 in, 2 out]
                  }
                }
                n99 = Index Array(array=w319) -> (element #1=w318:bool, element #2=w317:bool)  [unwired: 2 in]
                n100 = local write "0° M2"(w317) -> ()
                n101 = local write "0° M1"(w318) -> ()
              }
            }
          }
          event "stop": Value Change {
            n102 = event-data() -> ()  [unwired: 1 in, 1 out]
            n103 = local write "Ready"(FALSE ("READY 2")) -> ()
          }
          event "Move motors": Value Change {
            w352 = T7 1 items=["", "Forward", "Backward"] ("Direction motor 1")
            n104 = event-data() -> ()  [unwired: 1 in, 1 out]
            n105 = local read "Angulo M1"() -> (w350:dbl)
            "Angulo inicial" <- w350
            n106 = Unbundle By Name(w354) -> ("Arduino port"=w353:refnum<visa-resource-name>)
            n107 = Subtract(x="Ángulo final", y=w350) -> (x-y=w349:dbl)
            n108 = Multiply(x=w349, y=100.0) -> (x*y=w361:dbl)
            n109 = To Unsigned Word Integer(number=w361) -> (unsigned 16bit integer=w364:u16)
            n110 = property on="Real Time Measurement" class="XYGraph (strict)"(error in=w357, "XScale.Minimum"=w350, "XScale.Maximum"="Ángulo final", "Value"=cluster{"X":dbl, "X 2":dbl}[] []) -> (error out=w356:errorcluster)  [unwired: 1 in, 1 out]
            n111 = Multiply(x=w364, y=u16 2) -> (x*y=w362:u16)
            n112 = property on="Tab Control" class="TabCtl (strict)"("Value"=T3."Gráfica" ("Tab Control")) -> ()  [unwired: 2 in, 2 out]
            n113 = property on="Stop motors" class="Bool"("DisabledEnum"=T11."Enabled" ("Disabled")) -> ()  [unwired: 2 in, 2 out]
            n114 = Bundle By Name(cluster=T6 {"Action"=2, "Direction motor 1"=2, "Direction motor 2"=2, "Steps motor 1"=0, "Steps motor 2"=0, "Step style motor 1"=2, "Step style motor 2"=2} ("Comando"), "Steps motor 1"=w364, "Steps motor 2"=w362, "Direction motor 1"=w352, "Direction motor 2"=w352) -> (w365:T6)
            n115 = call-poly "Write.vi"("error in (no error)"=w356, "Comando"=w365, "VISA resource name"=w353) -> ("error out"=w345:errorcluster)  [unwired: 6 in, 2 out]
            n116 = Bundle By Name(cluster=w370, "Motor params"=w365) -> (w369:T5)
            n117 = Enqueue Element(queue=w343, element=cluster{"Ángulo M1":dbl, "Voltage":dbl}[] [] ("cluster"), error in (no error)=w345) -> (error out=w344:errorcluster)  [unwired: 1 in, 2 out]
            n118 = property on="Save" class="Bool (strict)"(error in=w344, "Value"=TRUE ("Guardar Datos")) -> (error out=w347:errorcluster)  [unwired: 1 in, 1 out]
            n119 = call "Create New File.vi"("error in"=w347) -> ("error out"=w358:errorcluster, "File Directory"=w359:T4)  [unwired: 9 in]
          }
          event "Realizar Análisis": Value Change {
            n120 = event-data() -> ()  [unwired: 1 in, 1 out]
            n121 = call "Brewster Angle Analysis.vi"("Open File"="Abrir Archivo", "q Starting   2"="q Inicial", "q Final"="q Final", "Do BA Analysis"="Realizar Análisis") -> ("No. de datos"=→"No. de Muestras":i32, "qR"=→"qR":dbl, "Curve width"=→"Ancho de Curva":dbl, "q  Middle"=→"q Medio":dbl, "Minimun Intensity"=→"Intensidad \nMínima":dbl, "Reflective Index"=→"Índice":dbl, "Curve"=→"Brewster Angle Analysis":cluster{"EJE X":dbl[], dbl[]}, "Maximum Intensity"=→"Intensidad \nMáxima":dbl)  [unwired: 4 in]
          }
          event "Abeles Brewster": Value Change {
            n122 = event-data() -> ()  [unwired: 1 in, 1 out]
            n123 = call "Abeles Brewster Analysis.vi"("Open Substrate File"="Abrir Archivo de Sustrato", "Open Film File"="Abrir Archivo de Película", "q Starting"="q Inicial 2", "q Final"="q Final  2", "Do AB Analysis"="Abeles Brewster", "calculate error"="calcular error", "Error (degrees)"="Error (Grados)") -> ("ángulo B valor medio"=→"ángulo B medio":dbl, "Film qB +error"=→"Película qB +error":dbl, "Film RI +error"=→"Película IR +error":dbl, "Substrate qB"=→"Sustrato qB":dbl, "Film qB"=→"Película qB":dbl, "Substrate RI"=→"Sustrato IR":dbl, "Film RI"=→"Película IR":dbl, "Curves"=→"Abeles Brewster Analysis":cluster{dbl[], dbl[]}[])  [unwired: 4 in, 1 out]
          }
          event Value Change {
            w415 = T7 2 items=["", "Forward", "Backward"] ("Direction motor 1")
            n124 = event-data() -> ()  [unwired: 1 in, 1 out]
            n125 = Unbundle By Name(w414) -> ("Arduino port"=w413:refnum<visa-resource-name>)
            n126 = Multiply(x="RESOLUCIÓN", y=100.0) -> (x*y=w418:dbl)
            n127 = To Unsigned Word Integer(number=w418) -> (unsigned 16bit integer=w417:u16)
            n128 = Bundle By Name(cluster=T6 {"Action"=2, "Direction motor 1"=1, "Direction motor 2"=2, "Steps motor 1"=0, "Steps motor 2"=0, "Step style motor 1"=2, "Step style motor 2"=2} ("Comando"), "Direction motor 1"=w415, "Steps motor 1"=w417) -> (w419:T6)
            n129 = call-poly "Write.vi"("error in (no error)"=w426, "Comando"=w419, "VISA resource name"=w413) -> ("error out"=w428:errorcluster)  [unwired: 6 in, 2 out]
            n130 = local write "0° M1"(FALSE ("0° M1")) -> ()
            n131 = Bundle By Name(cluster=w425, "Motor params"=w419, "Home?"=FALSE) -> (w424:T5)
          }
          event Value Change {
            w433 = T7 1 items=["", "Forward", "Backward"] ("Direction motor 1")
            n132 = event-data() -> ()  [unwired: 1 in, 1 out]
            n133 = local read "RESOLUCIÓN"() -> (w437:dbl)
            n134 = Unbundle By Name(w432) -> ("Arduino port"=w431:refnum<visa-resource-name>)
            n135 = Multiply(x=w437, y=100.0) -> (x*y=w436:dbl)
            n136 = To Unsigned Word Integer(number=w436) -> (unsigned 16bit integer=w435:u16)
            n137 = Bundle By Name(cluster=T6 {"Action"=2, "Direction motor 1"=2, "Direction motor 2"=2, "Steps motor 1"=0, "Steps motor 2"=0, "Step style motor 1"=2, "Step style motor 2"=2} ("Comando"), "Direction motor 1"=w433, "Steps motor 1"=w435) -> (w438:T6)
            n138 = call-poly "Write.vi"("error in (no error)"=w444, "Comando"=w438, "VISA resource name"=w431) -> ("error out"=w446:errorcluster)  [unwired: 6 in, 2 out]
            n139 = local write "0° M1"(FALSE ("0° M1")) -> ()
            n140 = Bundle By Name(cluster=w443, "Motor params"=w438, "Home?"=FALSE) -> (w442:T5)
          }
          event Value Change {
            w451 = T7 2 items=["", "Forward", "Backward"] ("Direction motor 2")
            n141 = event-data() -> ()  [unwired: 1 in, 1 out]
            n142 = local read "RESOLUCIÓN"() -> (w454:dbl)
            n143 = Unbundle By Name(w450) -> ("Arduino port"=w449:refnum<visa-resource-name>)
            n144 = Multiply(x=w454, y=100.0) -> (x*y=w456:dbl)
            n145 = To Unsigned Word Integer(number=w456) -> (unsigned 16bit integer=w453:u16)
            n146 = Bundle By Name(cluster=T6 {"Action"=2, "Direction motor 1"=2, "Direction motor 2"=1, "Steps motor 1"=0, "Steps motor 2"=0, "Step style motor 1"=2, "Step style motor 2"=2} ("Comando"), "Direction motor 2"=w451, "Steps motor 2"=w453) -> (w455:T6)
            n147 = call-poly "Write.vi"("error in (no error)"=w462, "Comando"=w455, "VISA resource name"=w449) -> ("error out"=w464:errorcluster)  [unwired: 6 in, 2 out]
            n148 = local write "0° M2"(FALSE ("0° M1")) -> ()
            n149 = Bundle By Name(cluster=w461, "Motor params"=w455, "Home?"=FALSE) -> (w460:T5)
          }
          event Value Change {
            w469 = T7 1 items=["", "Forward", "Backward"] ("Direction motor 2")
            n150 = event-data() -> ()  [unwired: 1 in, 1 out]
            n151 = local read "RESOLUCIÓN"() -> (w472:dbl)
            n152 = Unbundle By Name(w468) -> ("Arduino port"=w467:refnum<visa-resource-name>)
            n153 = Multiply(x=w472, y=100.0) -> (x*y=w474:dbl)
            n154 = To Unsigned Word Integer(number=w474) -> (unsigned 16bit integer=w471:u16)
            n155 = Bundle By Name(cluster=T6 {"Action"=2, "Direction motor 1"=2, "Direction motor 2"=2, "Steps motor 1"=0, "Steps motor 2"=0, "Step style motor 1"=2, "Step style motor 2"=2} ("Comando"), "Direction motor 2"=w469, "Steps motor 2"=w471) -> (w473:T6)
            n156 = call-poly "Write.vi"("error in (no error)"=w480, "Comando"=w473, "VISA resource name"=w467) -> ("error out"=w482:errorcluster)  [unwired: 6 in, 2 out]
            n157 = local write "0° M2"(FALSE ("0° M1")) -> ()
            n158 = Bundle By Name(cluster=w479, "Motor params"=w473, "Home?"=FALSE) -> (w478:T5)
          }
          event "Stop motors": Value Change {
            w489 = T11."Enabled" ("Disabled")
            n159 = event-data() -> ()  [unwired: 1 in, 1 out]
            n160 = Unbundle By Name(w484) -> ("Arduino port"=w483:refnum<visa-resource-name>)
            n161 = call "Stop.vi"("error in (no error)"=w494, "VISA resource name"=w483) -> ("error out"=w495:errorcluster)  [unwired: 8 in, 1 out]
            n162 = Bundle By Name(cluster=w492, "Moving?"=FALSE) -> (w491:T5)
            n163 = property on="Stop motors" class="Bool"("DisabledEnum"=T11."Disabled and Grayed Out" ("Disabled")) -> ()  [unwired: 2 in, 2 out]
            n164 = property on="Move motors" class="Bool"("DisabledEnum"=w489) -> ()  [unwired: 2 in, 2 out]
            n165 = property on="Home" class="Bool"("DisabledEnum"=w489) -> ()  [unwired: 2 in, 2 out]
            n166 = local write "Save"(FALSE ("Guardar Datos")) -> ()
          }
          event "Get position": Value Change {
            n167 = event-data() -> ()  [unwired: 1 in, 1 out]
            n168 = Unbundle By Name(w497) -> ("Arduino port"=w496:refnum<visa-resource-name>)
            n169 = Unbundle By Name(w507) -> ("Motor params"=w498:T6, "°/step"=w505:dbl[], "Motor positions"=w508:dbl[])
            n170 = call "Get position 2.vi"("Motor params"=w498, "°/step"=w505, "error in (no error)"=w512, "Positions in"=w508, "VISA resource name in"=w496) -> ("error out"=w509:errorcluster, "Positions out"=w504:dbl[])  [unwired: 4 in, 1 out]
            n171 = Bundle By Name(cluster=w507, "Motor positions"=w504) -> (w506:T5)
            n172 = Index Array(array=w504, index=0) -> (element=w501:dbl)
            n173 = Index Array(array=w504, index=1) -> (element=w500:dbl)
            n174 = local write "Angulo M1"(w501) -> ()
            n175 = local write "Angulo M2"(w500) -> ()
          }
          event "Read sensor": Value Change {
            n176 = event-data() -> ()  [unwired: 1 in, 1 out]
            n177 = Unbundle By Name(w514) -> ("Arduino port"=w513:refnum<visa-resource-name>)
            n178 = Unbundle By Name(w518) -> ("Sensor value"=w519:dbl)
            n179 = call "Read sensor 2.vi"("error in (no error)"=w523, "Sensor value in"=w519, "VISA resource name in"=w513) -> ("error out"=w520:errorcluster, "Sensor value out"=w516:dbl)  [unwired: 6 in, 1 out]
            n180 = Bundle By Name(cluster=w518, "Sensor value"=w516) -> (w517:T5)
            n181 = local write "Valor de Sensor"(w516) -> ()
          }
          event "Intensidad del Láser": Value Change {
            n182 = event-data() -> ()  [unwired: 1 in, 1 out]
            n183 = Unbundle By Name(w525) -> ("Arduino port"=w524:refnum<visa-resource-name>)
            n184 = call "Set Laser PWM.vi"("error in (no error)"=w531, "PWM Duty cycle"="Intensidad del Láser", "VISA Refnum in"=w524) -> ("error out"=w530:errorcluster)  [unwired: 7 in, 1 out]
          }
          event "Read End-stops": Value Change {
            n185 = event-data() -> ()  [unwired: 1 in, 1 out]
            n186 = Unbundle By Name(w534) -> ("Arduino port"=w533:refnum<visa-resource-name>)
            n187 = Unbundle By Name(w541) -> ("End-stop state"=w542:bool[])
            n188 = call "Read endstops.vi"("error in (no error)"=w543, "Ens-stop state in"=w542, "VISA Refnum in"=w533) -> ("error out"=w544:errorcluster, "Ens-stop state"=w538:bool[])  [unwired: 6 in, 1 out]
            n189 = Bundle By Name(cluster=w541, "End-stop state"=w538) -> (w540:T5)
            n190 = Index Array(array=w538) -> (element #1=w537:bool, element #2=w535:bool)  [unwired: 2 in]
            n191 = local write "0° M1"(w537) -> ()
            n192 = local write "0° M2"(w535) -> ()
          }
          event "Get all info": Value Change {
            n193 = event-data() -> ()  [unwired: 1 in, 1 out]
            n194 = Unbundle By Name(w547) -> ("Arduino port"=w546:refnum<visa-resource-name>)
            n195 = call "Get all info.vi"("error in (no error)"=w555, "VISA Refnum in"=w546) -> ("error out"=w554:errorcluster, "Recibo de Datos"=w552:string)  [unwired: 7 in, 1 out]
            "Recibo de Datos" <- w552
            n196 = call "Check info str.vi"("error in (no error)"=w554, "Data in"=w552, "Motor info"=w551) -> ("error out"=w553:errorcluster, "Motor info out"=w550:T5)  [unwired: 5 in, 2 out]
          }
          event "Home": Value Change {
            n197 = event-data() -> ()  [unwired: 1 in, 1 out]
            n198 = Unbundle By Name(w562) -> ("Motor positions"=w561:dbl[])
            n199 = call "Calculate Home direction.vi"("error in (no error)"=w560, "Motor positions"=w561) -> ("error out"=w559:errorcluster, "Home direction M2"=w558:T7, "Home direction M1"=w557:T7)  [unwired: 7 in]
            n200 = Unbundle By Name(w564) -> ("Arduino port"=w567:refnum<visa-resource-name>)
            n201 = call-poly "Write.vi"("error in (no error)"=w559, "Home direction (M2)"=w558, "Home direction (M1)"=w557, "VISA resource name"=w567) -> ("error out"=w563:errorcluster)  [unwired: 4 in, 3 out]
            n202 = Bundle By Name(cluster=w562, "Moving?"=TRUE, "Motor params.Direction motor 1"=w558, "Motor params.Direction motor 2"=w557) -> (w565:T5)
          }
          event "Velocidad del motor\n(0-255)": Value Change {
            n203 = event-data() -> ()  [unwired: 1 in, 1 out]
            n204 = Multiply(x="Velocidad del motor\n(0-255)", y=u16 2) -> (x*y=w573:u16)
            n205 = Bundle By Name(cluster=T12 {"Action"=1, "Steps per rev motor 1"=200, "Steps per rev motor 2"=200, "RPM motor 1"=100, "RPM motor 2"=200} ("Comando"), "RPM motor 1"="Velocidad del motor\n(0-255)", "RPM motor 2"=w573) -> (w580:T12)
            n206 = Unbundle By Name(w575) -> ("Arduino port"=w574:refnum<visa-resource-name>)
            n207 = call-poly "Write.vi"("error in (no error)"=w578, "Comando"=w580, "VISA resource name"=w574) -> ("error out"=w577:errorcluster)  [unwired: 6 in, 2 out]
          }
          event "Set zero": Value Change {
            n208 = event-data() -> ()  [unwired: 1 in, 1 out]
            n209 = Unbundle By Name(w590) -> ("Starting angle M1"=w589:dbl, "Starting angle M2"=w586:dbl)
            n210 = local read "Angulo M1"() -> (w588:dbl)
            n211 = local read "Angulo M2"() -> (w585:dbl)
            n212 = Add(x=w588, y=w589) -> (x+y=w587:dbl)
            n213 = Add(x=w586, y=w585) -> (x+y=w584:dbl)
            n214 = Bundle By Name(cluster=w590, "Starting angle M1"=w587, "Starting angle M2"=w584) -> (w592:T10)
          }
          event "Go to zero": Value Change {
            w597 = TRUE ("Moving?")
            w619 = T7 2 items=["", "Forward", "Backward"] ("f")
            w617 = T7 1 items=["", "Forward", "Backward"] ("Direction motor 1")
            w620 = T7 2 items=["", "Forward", "Backward"] ("f")
            w621 = T7 1 items=["", "Forward", "Backward"] ("Direction motor 1")
            n215 = event-data() -> ()  [unwired: 1 in, 1 out]
            n216 = Unbundle By Name(w603) -> ("Home?"=w598:bool, "Motor positions"=w631:dbl[])
            n217 = Unbundle By Name(w632) -> ("Arduino port"=w624:refnum<visa-resource-name>, "Starting angle M1"=w628:dbl, "Starting angle M2"=w626:dbl)
            n218 = Index Array(array=w631) -> (element #1=w629:dbl, element #2=w627:dbl)  [unwired: 2 in]
            n219 = local write "Idle"(FALSE ("Idle")) -> ()
            n220 = case shown="True" w598 {
              tunnel: w629 -> [w638 w644]
              tunnel: w628 -> [_ w643]
              tunnel: w627 -> [w635 w642]
              tunnel: w626 -> [_ w641]
              tunnel: [w637 w640] -> w613
              tunnel: [w636 w639] -> w612
              frame False {
                n221 = Negate(x=w638) -> (-x=w637:dbl)
                n222 = Negate(x=w635) -> (-x=w636:dbl)
              }
              frame True {
                n223 = Subtract(x=w643, y=w644) -> (x-y=w640:dbl)
                n224 = Subtract(x=w641, y=w642) -> (x-y=w639:dbl)
              }
            }
            n225 = Greater Or Equal To 0?(x=w613) -> (x >= 0?=w622:bool)
            n226 = Greater Or Equal To 0?(x=w612) -> (x >= 0?=w618:bool)
            n227 = Select(t=w621, s=w622, f=w620) -> (s? t:f=w616:T7)
            n228 = Absolute Value(x=w613) -> (abs(x)=w614:dbl)
            n229 = Absolute Value(x=w612) -> (abs(x)=w611:dbl)
            n230 = Select(t=w617, s=w618, f=w619) -> (s? t:f=w615:T7)
            n231 = To Unsigned Word Integer(number=w611) -> (unsigned 16bit integer=w610:u16)
            n232 = To Unsigned Word Integer(number=w614) -> (unsigned 16bit integer=w606:u16)
            n233 = Multiply(x=u16 100 ("y"), y=w606) -> (x*y=w607:u16)
            n234 = Multiply(x=w610, y=u16 100) -> (x*y=w609:u16)
            n235 = Bundle By Name(cluster=T6 {"Action"=2, "Direction motor 1"=1, "Direction motor 2"=2, "Steps motor 1"=0, "Steps motor 2"=0, "Step style motor 1"=2, "Step style motor 2"=2} ("Comando"), "Direction motor 1"=w616, "Steps motor 1"=w607, "Direction motor 2"=w615, "Steps motor 2"=w609) -> (w601:T6)
            n236 = property on="Go to zero" class="Bool"("DisabledEnum"=T11."Disabled and Grayed Out" ("Disabled")) -> ()  [unwired: 2 in, 2 out]
            n237 = Bundle By Name(cluster=w603, "Moving?"=w597, "Manual zero?"=w597, "Motor params"=w601) -> (w602:T5)
            n238 = call-poly "Write.vi"("error in (no error)"=w599, "Comando"=w601, "VISA resource name"=w624) -> ("error out"=w623:errorcluster)  [unwired: 6 in, 2 out]
          }
        }
      }
      frame "Configuration dialog" {
        n239 = call "COM Port selector español.vi"() -> ("Cancelled?"=w646:bool, "VISA Refnum out"=w649:refnum<visa-resource-name>)  [unwired: 10 in]
        n240 = case shown="False" w646 {
          tunnel: w651 -> [w660 w662]
          tunnel: [w659 w662] -> w650
          tunnel: w649 -> [w658 _]
          tunnel: [w657 w661] -> w648
          tunnel: w647 -> [w656 w661]
          tunnel: [States_--_typedef."Initilaize" ("Unused") States_--_typedef."Wait" ("Unused")] -> w645
          frame False {
            # "File dialog not cancelled. Apply new config."
            n241 = Bundle By Name(cluster=w656, "Arduino port"=w658) -> (w657:T10)
            n242 = call "Save config.vi"("error in (no error)"=w660, "Config"=w657) -> ("error out"=w659:errorcluster)  [unwired: 9 in]
          }
          frame True {
            # "File dialog cancelled. Do nothing."
          }
        }
      }
      frame "Update config" {
        n243 = local write "Angulo M1"(0.0 ("Angulo M1")) -> ()
        n244 = local write "Angulo M2"(0.0 ("Angulo M2")) -> ()
        n245 = call "Save config.vi"("error in (no error)"=w673, "Config"=w671) -> ("error out"=w672:errorcluster)  [unwired: 9 in]
        n246 = Bundle By Name(cluster=w666, "Motor positions"=dbl[] [0.0, 0.0]) -> (w665:T5)
      }
      frame "Update FP" {
        n247 = Unbundle By Name(w697) -> ("Motor positions"=w685:dbl[], "Sensor value"=w687:dbl, "End-stop state"=w695:bool[])
        "Valor de Sensor" <- w687
        n248 = Index Array(array=w695) -> (element #1=→"0° M1":bool, element #2=→"0° M2":bool)  [unwired: 2 in]
        n249 = Unbundle By Name(w693) -> ("refnum out"=w691:refnum<file>)
        n250 = local read "Ángulo final"() -> (w684:dbl)
        n251 = Index Array(array=w685) -> (element #1=w683:dbl, element #2=→"Angulo M2":dbl)  [unwired: 2 in]
        "Angulo M1" <- w683
        n252 = Subtract(x=w684, y=w683) -> (x-y=w682:dbl)
        n253 = local read "Save"() -> (w678:bool)
        n254 = In Range and Coerce(upper limit=0.1, x=w682, lower limit=-0.1) -> (In Range?=w679:bool)  [unwired: 1 out]
        n255 = Not(x=w679) -> (.not. x?=w676:bool)
        n256 = And(x=w678, y=w676) -> (x .and. y?=w677:bool)
        n257 = case shown="False" w677 {
          selector: w677 -> [_ w708]
          tunnel: w675 -> [_ w711]
          tunnel: [w699 w710] -> w692
          tunnel: w691 -> [_ w709]
          tunnel: w690 -> [w699 w706]
          tunnel: w687 -> [_ w704]
          tunnel: w683 -> [_ w702]
          tunnel: w683 -> [_ w701]
          frame False {
            # "Final angle has been achieved to a certain tolerance. Stop saving and updating graph."
            n258 = local write "Save"(FALSE ("Save")) -> ()
          }
          frame True {
            # "Save flag is set and angle difference is still big. Save data and update graph."
            n259 = call "Save Graph Data.vi"("refnum in"=w709, "Save Data Enable"=w708, "Optic Sensor Data"=w704, "Degrees"=w701, "error in"=w706) -> ("error out"=w707:errorcluster)  [unwired: 9 in, 1 out]
            n260 = Bundle(cluster=cluster{"Ángulo M1":dbl, "Voltage":dbl} {"Ángulo M1"=0.0, "Voltage"=0.0}, "Ángulo M1"=w702, "Voltage"=w704) -> (w703:cluster{"Ángulo M1":dbl, "Voltage":dbl})
            n261 = Enqueue Element(queue=w711, element=w703, error in (no error)=w707) -> (error out=w710:errorcluster)  [unwired: 1 in, 2 out]
          }
        }
      }
      frame "Enable/disable controls" {
        n262 = Unbundle By Name(w715) -> ("Moving?"=w714:bool, "Home?"=w713:bool)
        n263 = case shown="False" w714 {
          tunnel: w713 -> [w725 _]
          frame False {
            w721 = T11."Disabled and Grayed Out" ("Disabled")
            w720 = T11."Enabled" ("Disabled")
            # "Device not moving or home reached. Check stop condition."
            n264 = property on="Move motors" class="Bool"("DisabledEnum"=w720) -> ()  [unwired: 2 in, 2 out]
            n265 = property on="CW Button M1" class="Bool"("DisabledEnum"=w720) -> ()  [unwired: 2 in, 2 out]
            n266 = property on="CW Button M2" class="Bool"("DisabledEnum"=w720) -> ()  [unwired: 2 in, 2 out]
            n267 = property on="CCW Button M1" class="Bool"("DisabledEnum"=w720) -> ()  [unwired: 2 in, 2 out]
            n268 = property on="CCW Button M2" class="Bool"("DisabledEnum"=w720) -> ()  [unwired: 2 in, 2 out]
            n269 = property on="Set zero" class="Bool"("DisabledEnum"=w720) -> ()  [unwired: 2 in, 2 out]
            n270 = Not(x=w725) -> (.not. x?=w723:bool)
            n271 = Select(t=w721, s=w725, f=w720) -> (s? t:f=w722:T11)
            n272 = Select(t=w721, s=w723, f=w720) -> (s? t:f=w724:T11)
            n273 = property on="Stop motors" class="Bool"("DisabledEnum"=w721) -> ()  [unwired: 2 in, 2 out]
            n274 = property on="Home" class="Bool"("DisabledEnum"=w722) -> ()  [unwired: 2 in, 2 out]
            n275 = property on="Move motors" class="Bool"("DisabledEnum"=w724) -> ()  [unwired: 2 in, 2 out]
          }
          frame True {
            w726 = T11."Disabled and Grayed Out" ("Disabled")
            # "Device is moving. Disable all moving commands."
            n276 = property on="Stop motors" class="Bool"("DisabledEnum"=T11."Enabled" ("Disabled")) -> ()  [unwired: 2 in, 2 out]
            n277 = property on="Home" class="Bool"("DisabledEnum"=w726) -> ()  [unwired: 2 in, 2 out]
            n278 = property on="Set zero" class="Bool"("DisabledEnum"=w726) -> ()  [unwired: 2 in, 2 out]
            n279 = property on="CW Button" class="Bool"("DisabledEnum"=w726) -> ()  [unwired: 2 in, 2 out]
            n280 = property on="CW Button" class="Bool"("DisabledEnum"=w726) -> ()  [unwired: 2 in, 2 out]
            n281 = property on="Motor 2 Backward Button" class="Bool"("DisabledEnum"=w726) -> ()  [unwired: 2 in, 2 out]
            n282 = property on="Motor 2 Forward Button" class="Bool"("DisabledEnum"=w726) -> ()  [unwired: 2 in, 2 out]
            n283 = property on="Move motors" class="Bool"("DisabledEnum"=w726) -> ()  [unwired: 2 in, 2 out]
          }
        }
      }
      frame "Exit" {
        w735 = States_--_typedef."Wait"  # Unused
        n284 = Unbundle By Name(w729) -> ("Connected?"=w728:bool)
        n285 = case shown="True" w728 {
          tunnel: w733 -> [w737 w746]
          tunnel: [w737 w743] -> w732
          tunnel: w730 -> [_ w739]
          frame False {
          }
          frame True {
            w744 = u8 1  # Duty cycle
            n286 = Unbundle By Name(w739) -> ("Arduino port"=w738:refnum<visa-resource-name>)
            n287 = call "Stop.vi"("error in (no error)"=w746, "VISA resource name"=w738) -> ("error out"=w742:errorcluster, "VISA resource name out"=w745:refnum<visa-resource-name>)  [unwired: 8 in]
            n288 = call "Wait -- constant.vi"("wait (200 ms)"=u32 300, "error in (no error)"=w742) -> ("error out"=w741:errorcluster)  [unwired: 3 in]
            n289 = call "Set Laser PWM.vi"("error in (no error)"=w741, "PWM Duty cycle"=w744, "VISA Refnum in"=w745) -> ("error out"=w743:errorcluster)  [unwired: 7 in, 1 out]
          }
        }
      }
    }
    n290 = Or(x=w45, y=w46) -> (x .or. y?=w39:bool)
  }
  n291 = Unbundle By Name(w7) -> ("Arduino port"=w6:refnum<visa-resource-name>)
  n292 = Unbundle By Name(w2) -> ("Connected?"=w1:bool)
  n293 = case shown="True" w1 {
    tunnel: w17 -> [w747 w751]
    tunnel: [w747 w753] -> w10
    tunnel: w6 -> [_ w752]
    frame False {
    }
    frame True {
      n294 = call <vilib>:"Clear Errors.vi"("error in (no error)"=w751, "specific error code to clear (0: all)"=1) -> ("error out"=w750:errorcluster, "specific error cleared?"=w748:bool)  [unwired: 4 in]
      n295 = case shown="True" w748 {
        frame False {
        }
        frame True {
          n296 = One Button Dialog(message="Se produjo un error inesperado. Cerrando comunicaciones.") -> ()  [unwired: 1 in, 1 out]
        }
      }
      n297 = call "Close.vi"("error in (no error)"=w750, "VISA resource name"=w752) -> ("error out"=w753:errorcluster)  [unwired: 9 in]
    }
  }
  n298 = Release Queue(queue=w11, error in (no error)=w10) -> (error out=w8:errorcluster)  [unwired: 1 in, 2 out]
  n299 = disable-structure shown="Default" {
    disable-tunnel: w8 -> [w755 _]
    frame condition #0 (active) {
      n300 = call <vilib>:"Simple Error Handler.vi"("error in (no error)"=w755) -> ()  [unwired: 4 in, 5 out]
    }
    frame condition #1 {
      n301 = Quit LabVIEW() -> ()  [unwired: 1 in]
    }
  }
